vi "wait for temp to settle.vi"(5 "Current setpoint":dbl format="%.2f", 7 "Timing Control Parameters In":T1={"N cycles for averaging"=30, "N points per measurement"=1000, "Measurment time interval"=2e-05} {"Measurment time interval" format="%.2e"}, 11 "error in":errorcluster) -> (8 "Timing Control Parameters Out":T1={"N cycles for averaging"=30, "N points per measurement"=1000, "Measurment time interval"=2e-05} {"Measurment time interval" format="%.2e"}, 15 "error out":errorcluster)   [LabVIEW 2014]
doc: "wait for temp to settle\n\nUpdates the control setpoint and waits until the temperature reaches the setpoint, while considering changes from executive stop, error detection, and early proceed.\n\nBeverly Abadines \nPHY 350\nP6"
uses:
  temp control/globals/temp control global variables.vi
  globals/C(T) global variables.vi
panel:
  out "time in this wait cycle (sec)":dbl format="%.1f"
  in  "Proceed":bool
  # "C(T) Waiting for Temp to settle"
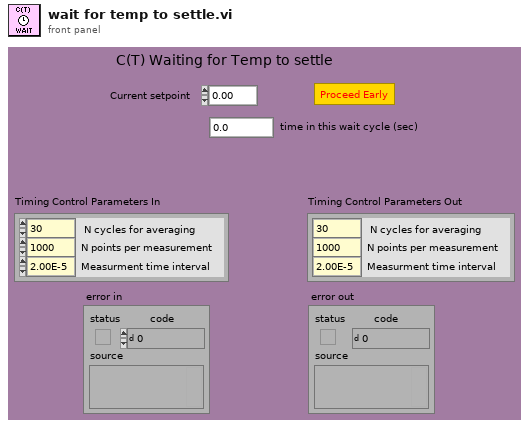
[diagram p1: front panel]
types:
  T1 = cluster{"N cycles for averaging":i32, "N points per measurement":i32, "Measurment time interval":dbl}
  T2 = typedef "control parameters.ctl" = cluster{"Setpoint":dbl, "Control bandwidth":dbl, "Settle bandwidth":dbl, "Integral time":dbl, "Int\non":bool, "Derivative time":dbl, "Der\non":bool, "Settle time":dbl}
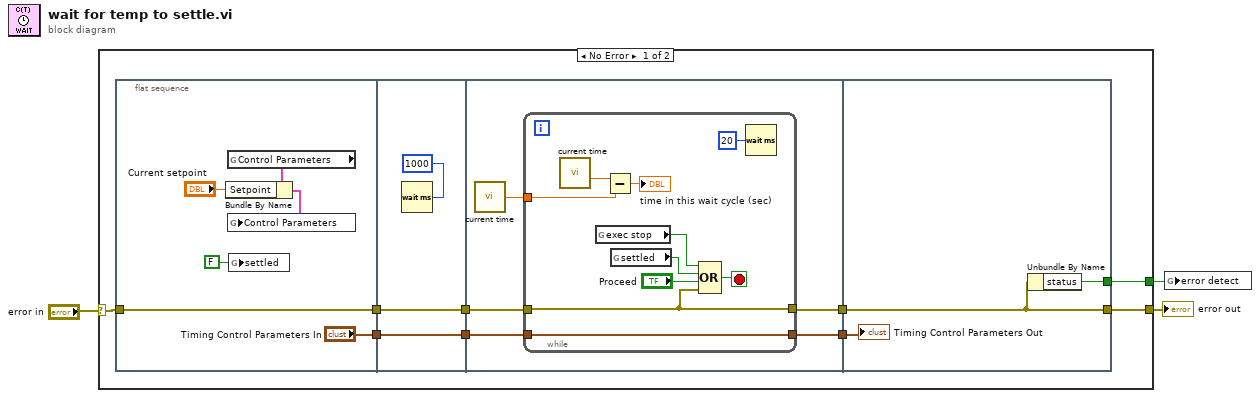
[diagram p0: block diagram]
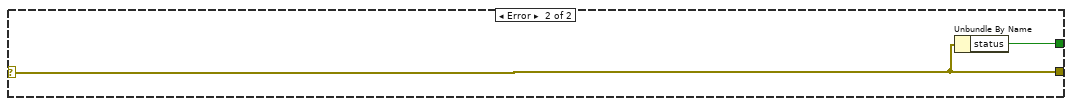
[diagram p2: hidden frame]
diagram:
  n1 = case shown="No Error" "error in" {
    selector: "error in" -> [w12 w41]
    tunnel: [w5 w41] -> w2
    tunnel: [w4 w40] -> w1
    frame No Error {
      n2 = flat-sequence {
        tunnel: w12 -> [w16]
        tunnel: [w16] -> w10
        tunnel: ["Timing Control Parameters In"] -> w7
        tunnel: w10 -> [w21]
        tunnel: [w21] -> w9
        tunnel: [w19] -> w8
        tunnel: w7 -> [w19]
        tunnel: w9 -> [w26]
        tunnel: [w25] -> w11
        tunnel: w8 -> [w24]
        tunnel: [w23] -> w6
        tunnel: w11 -> [w38]
        tunnel: [w38] -> w5
        tunnel: w6 -> [w39]
        tunnel: [w37] -> w4
        frame #0 {
          n3 = global read "temp control global variables.vi" "Control Parameters"() -> (w18:T2)
          n4 = Bundle By Name(cluster=w18, "Setpoint"="Current setpoint") -> (w15:T2)
          n5 = global write "temp control global variables.vi" "Control Parameters"(w15) -> ()
          n6 = global write "temp control global variables.vi" "settled"(FALSE ("settled")) -> ()
        }
        frame #1 {
          n7 = Wait (ms)(milliseconds to wait=u32 1000) -> ()  [unwired: 1 out]
        }
        frame #2 {
          n8 = call "current time.vi"() -> ("current time (sec)"=w22:dbl)
          n9 = while {
            tunnel: w26 -> [w35]
            tunnel: [w35] -> w25
            tunnel: w24 -> [w34]
            tunnel: [w34] -> w23
            tunnel: w22 -> [w32]
            stop <- w36 stop-if-true
            n10 = call "current time.vi"() -> ("current time (sec)"=w33:dbl)
            n11 = global read "C(T) global variables.vi" "exec stop"() -> (w31:bool)
            n12 = Subtract(x=w33, y=w32) -> (x-y=→"time in this wait cycle (sec)":dbl)
            n13 = global read "temp control global variables.vi" "settled"() -> (w28:bool)
            n14 = Compound Arithmetic op=OR(w31, w28, "Proceed", w35) -> (w36:bool)
            n15 = Wait (ms)(milliseconds to wait=u32 20) -> ()  [unwired: 1 out]
          }
        }
        frame #3 {
          n16 = Unbundle By Name(w38) -> ("status"=w37:bool)
          "Timing Control Parameters Out" <- w39
        }
      }
    }
    frame Error {
      n17 = Unbundle By Name(w41) -> ("status"=w40:bool)
    }
  }
  "error out" <- w2
  n18 = global write "C(T) global variables.vi" "error detect"(w1) -> ()
